vi "FTCU Adjust.vi"(8 "error in":errorcluster, 11 "DAC FTCU in":refnum<class "DAC FTCU.lvclass">) -> (0 "error out":errorcluster, 3 "DAC FTCU out":refnum<class "DAC FTCU.lvclass">)   [LabVIEW 2019, in "DAC.lvlib" / "DAC FTCU.lvclass"]
uses:
  DAC FTCU.lvclass
  Results/Results Method.ctl
  Results/DeepU Results/DeepU Results.lvclass
  DAC FTCU.lvclass/DAC FTCU.ctl
  Results/DeepU Results/DeepU Results.lvclass/DeepU Results.ctl
  <vilib>/NI/Modbus Library/API/Master/Modbus Master.lvclass
  Results/Results.lvlib
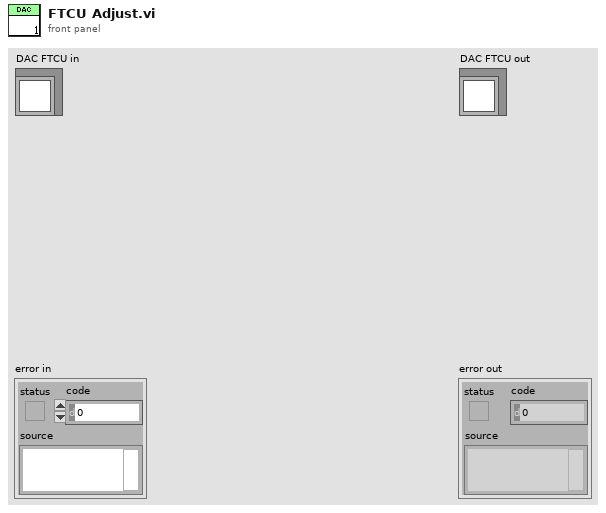
[diagram p1: front panel]
types:
  T1 = typedef "Results.lvlib/Results Method.ctl" = enum16{"Get", "Set"}
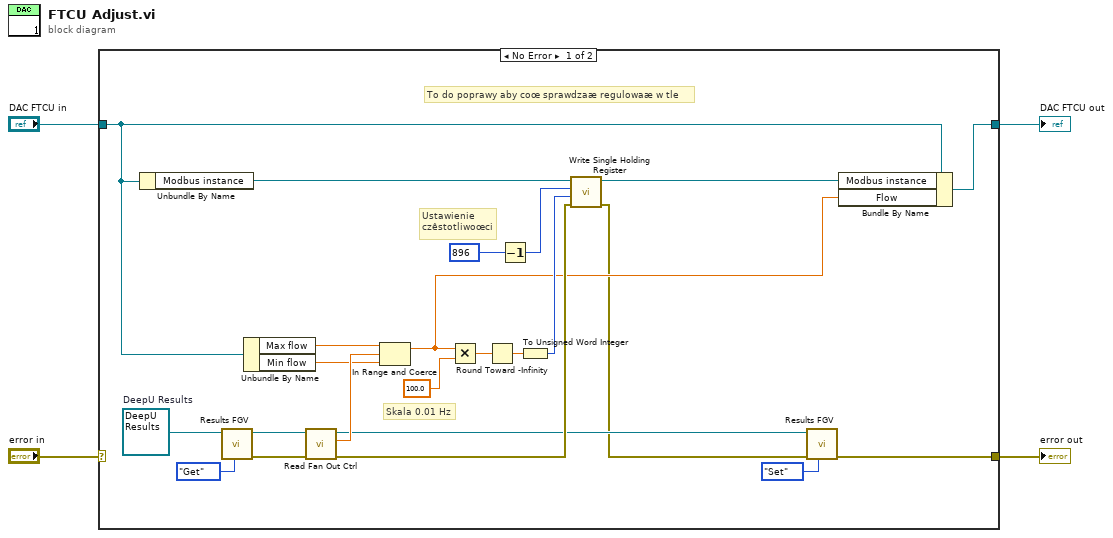
[diagram p0: block diagram]
diagram:
  n1 = case shown="No Error" "error in" {
    selector: "error in" -> [_ w29]
    tunnel: [w5 w29] -> w3
    tunnel: [w21 w28] -> w1
    tunnel: "DAC FTCU in" -> [w15 w28]
    frame No Error {
      w27 = refnum<class "DeepU Results.lvclass"> refnum  # DeepU Results
      # "To do poprawy aby coœ sprawdzaæ regulowaæ w tle"
      # "Skala 0.01 Hz"
      # "Ustawienie\nczêstotliwoœci"
      n2 = Unbundle By Name(w15) -> ("Modbus instance"=w22:refnum<class "Modbus Master.lvclass">)
      n3 = call-dynamic "Results FGV.vi"("Method"=Results_Method."Get", "DeepU Results in"=w27) -> ("error out"=w18:errorcluster, "DeepU Results out"=w19:refnum<class "DeepU Results.lvclass">)  [unwired: 8 in]
      n4 = Unbundle By Name(w15) -> ("Max flow"=w14:dbl, "Min flow"=w13:dbl)
      n5 = call "Read Fan Out Ctrl.vi"("error in (no error)"=w18, "DeepU Results in"=w19) -> ("error out"=w9:errorcluster, "Fan Out Ctrl"=w16:dbl, "DeepU Results out"=w7:refnum<class "DeepU Results.lvclass">)  [unwired: 7 in]
      n6 = In Range and Coerce(upper limit=w14, x=w16, lower limit=w13) -> (coerced(x)=w8:dbl)  [unwired: 1 out]
      n7 = Multiply(x=w8, y=100.0) -> (x*y=w12:dbl)
      n8 = Round Toward -Infinity(1:w12) -> (0:w11:dbl)
      n9 = Decrement(x=u16 896 ("address")) -> (x-1=w23:u16)
      n10 = To Unsigned Word Integer(number=w11) -> (unsigned 16bit integer=w10:u16)
      n11 = call-dynamic "Write Single Holding Register.vi"("error in"=w9, "register to write"=w10, "address"=w23, "Modbus master in"=w22) -> ("error out"=w6:errorcluster, "Modbus master out"=w20:refnum<class "Modbus Master.lvclass">)  [unwired: 6 in]
      n12 = call-dynamic "Results FGV.vi"("Method"=Results_Method."Set", "error in"=w6, "DeepU Results in"=w7) -> ("error out"=w5:errorcluster)  [unwired: 7 in, 1 out]
      n13 = Bundle By Name(cluster=w15, "Modbus instance"=w20, "Flow"=w8) -> (w21:refnum<class "DAC FTCU.lvclass">)
    }
    frame Error {
    }
  }
  "error out" <- w3
  "DAC FTCU out" <- w1
